vi "Get SubPnl Ref.vi"(11 "Series Actor in":refnum<class "Series Actor.lvclass">) -> (2 "SubPnl Ref":refnum<vi>, 3 "Series Actor out":refnum<class "Series Actor.lvclass">)   [LabVIEW 2024, in "Series Actor.lvlib" / "Series Actor.lvclass"]
uses:
  Series Actor.lvclass
  Series Actor.lvclass/Series Actor.ctl
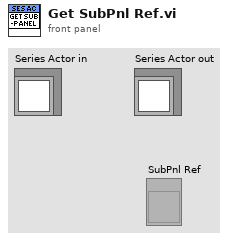
[diagram p1: front panel]
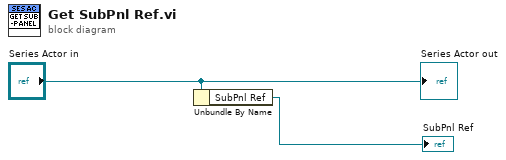
[diagram p0: block diagram]
diagram:
  n1 = Unbundle By Name("Series Actor in") -> ("SubPnl Ref"=→"SubPnl Ref":refnum<vi>)
  "Series Actor out" <- "Series Actor in"
